vi "FTW-Subscription-Worker.vi"(1 "Endpoint":refnum<class "FTW-Endpoint.lvclass">, 2 "Message Handler":refnum<user-event>) -> ()   [LabVIEW 2013, in "FTW-Subscription.lvclass"]
uses:
  FTW-Subscription.lvclass
  Message/Base/FTW-Message.lvclass
  Endpoint/FTW-Endpoint.lvclass
panel:
  out "Messages Received":u32
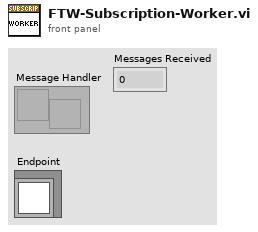
[diagram p1: front panel]
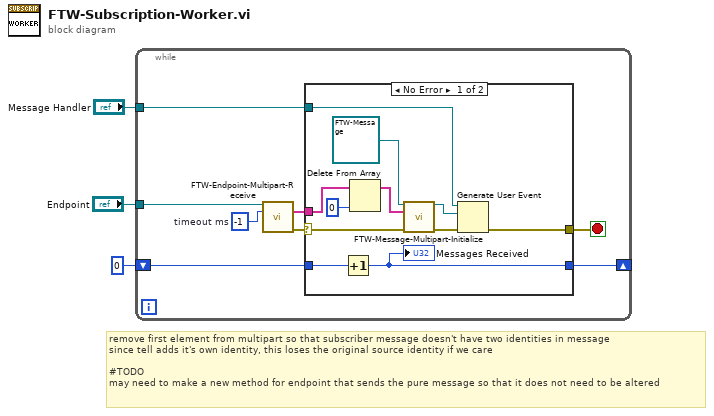
[diagram p0: block diagram]
diagram:
  # "remove first element from multipart so that subscriber message doesn't have two identities in message\nsince tell adds it's own identity, this loses the original source identity if we care\n\n#TODO\nmay need to make a new method for endpoint that sends the pure message so that it does not need to be altered"
  n1 = while {
    tunnel: "Message Handler" -> [w11]
    shift-right: [w5] -> _
    shift-left: u32 0 -> [w6]
    tunnel: "Endpoint" -> [w10]
    stop <- w7 stop-if-true
    w9 = -1  # timeout ms
    n2 = call-dynamic "FTW-Endpoint-Multipart-Receive.vi"("FTW Endpoint"=w10, "Timeout"=w9) -> ("Message Received"=w4:string[], "error out"=w8:errorcluster)  [unwired: 10 in, 2 out]
    n3 = case shown="No Error" w8 {
      selector: w8 -> [w21 w24]
      tunnel: w11 -> [w22 _]
      tunnel: w4 -> [w13 _]
      tunnel: [w20 w24] -> w7
      tunnel: w6 -> [w19 w23]
      tunnel: [w18 w23] -> w5
      frame No Error {
        n4 = Increment(x=w19) -> (x+1=w18:u32)
        "Messages Received" <- w18
        n5 = Delete From Array(array=w13, index=0) -> (array with subset deleted=w14:string[])  [unwired: 1 in, 1 out]
        n6 = call-dynamic "FTW-Message-Multipart-Initialize.vi"("FTW Message"=refnum<class "FTW-Message.lvclass"> refnum, "Message Parts"=w14, "error in"=w21) -> ("FTW Message out"=w16:refnum<class "FTW-Message.lvclass">, "error out"=w17:errorcluster)  [unwired: 11 in]
        n7 = Generate User Event(user event=w22, event data cluster=w16, error in=w17) -> (error out=w20:errorcluster)  [unwired: 1 in, 1 out]
      }
      frame Error {
      }
    }
  }
